vi "ROS_Master_getTopicTypesReply.vi"(3 "ROS_Master in":T1) -> (0 "Topics XML":string)   [LabVIEW 2015]
doc: "Returns XML replys from a topic"
uses:
  ROS_Master.ctl
  ROS_Topic.ctl
  ROS_Node.ctl
  ROS_Service.ctl
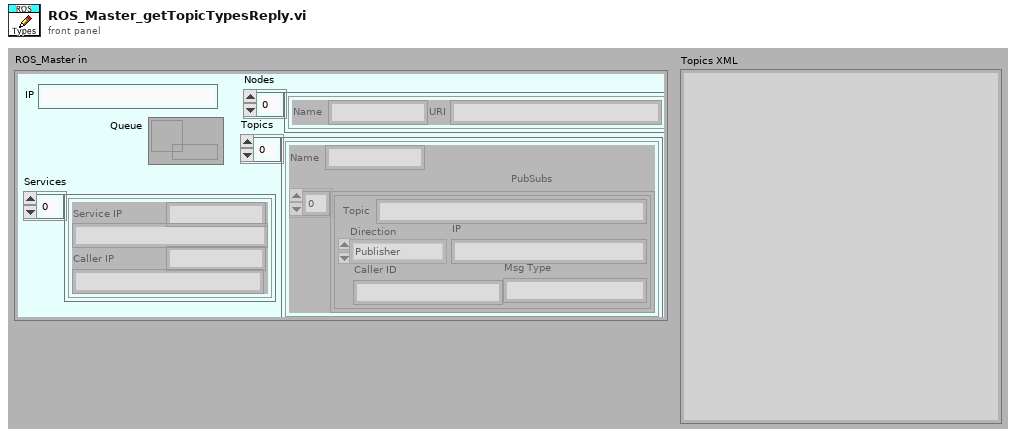
[diagram p1: front panel]
types:
  T1 = typedef "ROS_Master.ctl" = cluster{"IP":string, "Topics":cluster{"Name":string, "PubSubs":T2[]}[], "Nodes":T3[], "Services":T4[], "Queue":refnum<queue>}
  T2 = typedef "ROS_Topic.ctl" = cluster{"Caller ID":string, "IP":string, "Msg Type":string, "Direction":enum16{"Publisher", "Subscriber"}, "Topic":string}
  T3 = typedef "ROS_Node.ctl" = cluster{"Name":string, "URI":string}
  T4 = typedef "ROS_Service.ctl" = cluster{"Service":string, "Service IP":string, "Caller IP":string, "Caller ID":string}
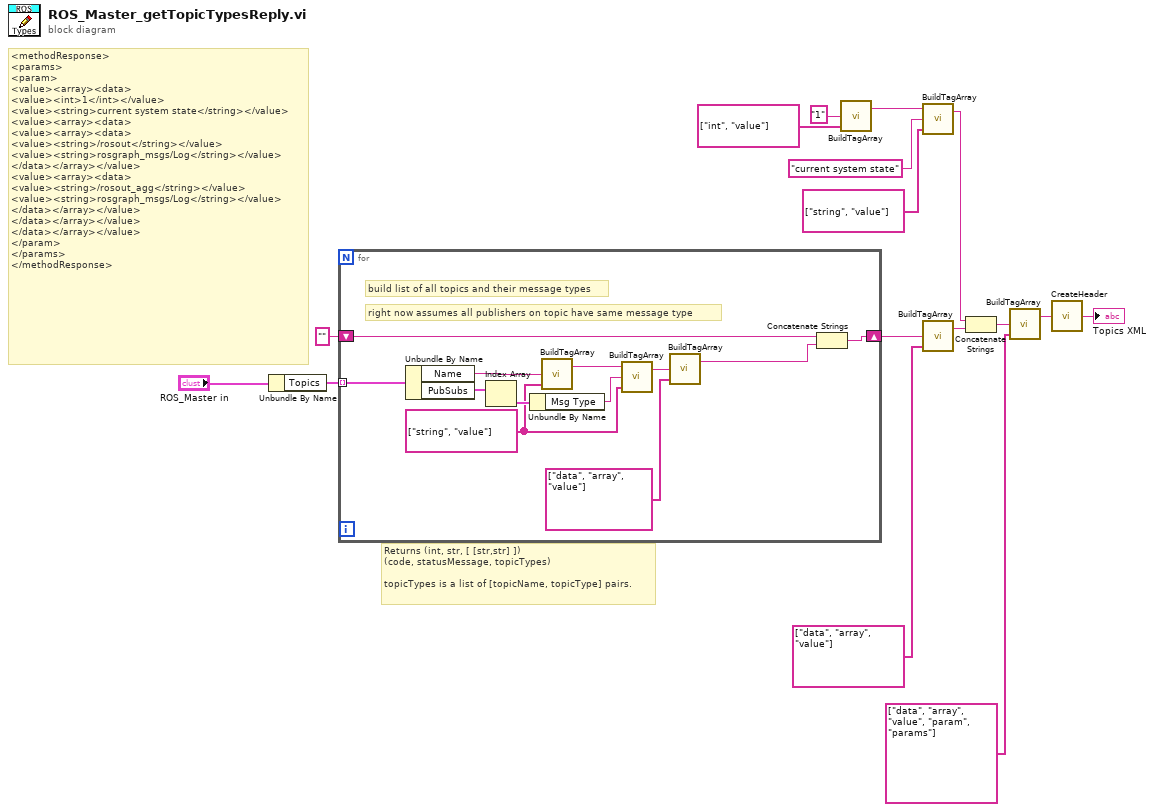
[diagram p0: block diagram]
diagram:
  # "<methodResponse>\n<params>\n<param>\n<value><array><data>\n<value><int>1</int></value>\n<value><string>current system state</string></value>\n<value><array><data>\n<value><array><data>\n<value><string>/rosout</string></value>\n<value><string>rosgraph_msgs/Log</string></value>\n</data></array></value>\n<value><array><data>\n<value><string>/rosout_agg</string></value>\n<value><string>rosgraph_msgs/Log</string></value>\n</data></array></value>\n</data></array></value>\n</data></array></value>\n</param>\n</params>\n</methodResponse>"
  # "Returns (int, str, [ [str,str] ])\n(code, statusMessage, topicTypes)\n\ntopicTypes is a list of [topicName, topicType] pairs."
  n1 = Unbundle By Name("ROS_Master in") -> ("Topics"=w2:cluster{"Name":string, "PubSubs":T2[]}[])
  n2 = for {
    tunnel: w2 -> [w28] mode=indexing
    shift-right: [w26] -> w9
    shift-left: "" ("string out") -> [w27]
    w21 = string[] ["string", "value"] ("tags")
    # "right now assumes all publishers on topic have same message type"
    # "build list of all topics and their message types"
    n3 = Unbundle By Name(w28) -> ("Name"=w25:string, "PubSubs"=w24:T2[])
    n4 = Index Array(array=w24) -> (element=w23:T2)  [unwired: 1 in]
    n5 = Unbundle By Name(w23) -> ("Msg Type"=w17:string)
    n6 = call "BuildTagArray.vi"("tags"=w21, "value"=w25) -> ("string out"=w22:string)  [unwired: 2 in]
    n7 = call "BuildTagArray.vi"("tags"=w21, "value"=w17, "string in"=w22) -> ("string out"=w20:string)  [unwired: 1 in]
    n8 = call "BuildTagArray.vi"("tags"=string[] ["data", "array", "value"], "value"=w20) -> ("string out"=w18:string)  [unwired: 2 in]
    n9 = Concatenate Strings(w27, w18) -> (w26:string)
  }
  n10 = call "BuildTagArray.vi"("tags"=string[] ["int", "value"], "value"="1") -> ("string out"=w11:string)  [unwired: 2 in]
  n11 = call "BuildTagArray.vi"("tags"=string[] ["string", "value"], "value"="current system state", "string in"=w11) -> ("string out"=w10:string)  [unwired: 1 in]
  n12 = call "BuildTagArray.vi"("tags"=string[] ["data", "array", "value"], "value"=w9) -> ("string out"=w8:string)  [unwired: 2 in]
  n13 = Concatenate Strings(w10, w8) -> (w7:string)
  n14 = call "BuildTagArray.vi"("tags"=string[] ["data", "array", "value", "param", "params"], "value"=w7) -> ("string out"=w4:string)  [unwired: 2 in]
  n15 = call "CreateHeader.vi"("Content"=w4) -> ("XML"=→"Topics XML":string)
